vi "On Go (SubVI).vi"(0 "CmdLib Out":refnum<k24>, 1 "Device Key":string, 2 "Relative Steps":i32, 3 "Motor":i32, 4 "Device Address":i32, 5 "error in":errorcluster) -> (19 "error out":errorcluster)   [LabVIEW 2017]
uses:
  dll/CmdLib.dll
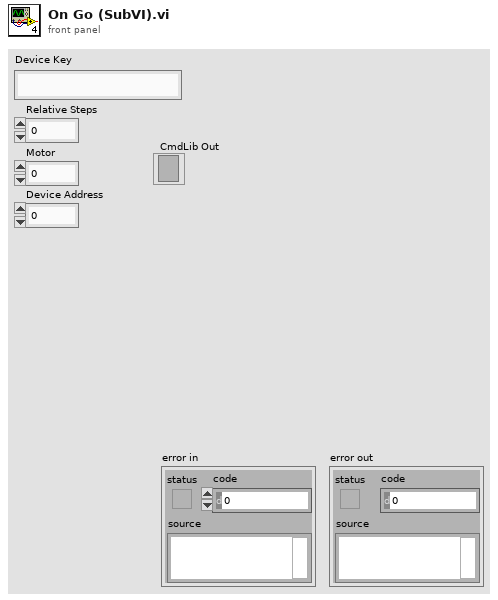
[diagram p1: front panel]
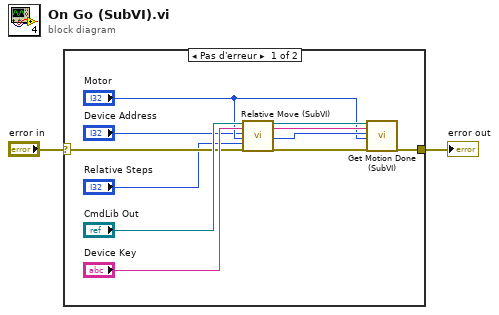
[diagram p0: block diagram]
diagram:
  n1 = case shown="Pas d'erreur" "error in" {
    selector: "error in" -> [w7 w14]
    tunnel: [w3 w14] -> w2
    frame No Error {
      n2 = call "Relative Move (SubVI).vi"("CmdLib In"="CmdLib Out", "DeviceKey In"="Device Key", "Device Address In"="Device Address", "Motor"="Motor", "Relative Steps"="Relative Steps", "error in (no error)"=w7) -> ("CmdLib Out"=w11:refnum<k24>, "DeviceKey Out"=w12:string, "Device Address Out"=w13:i32, "error out"=w10:errorcluster)  [unwired: 10 in]
      n3 = call "Get Motion Done (SubVI).vi"("CmdLib In"=w11, "DeviceKey In"=w12, "Device Address In"=w13, "Motor"="Motor", "error in (no error)"=w10) -> ("error out"=w3:errorcluster)  [unwired: 10 in, 4 out]
    }
    frame Error {
    }
  }
  "error out" <- w2
